vi "Sub_Online_FEA_Model.vi"(4 "Pin Location":i32, 11 "Modeling Parameters":T1) -> (2 "K Matrix":dbl[][](array[numeric]), 3 "M Matrix":dbl[][](array[numeric]))   [LabVIEW 2021]
panel:
  out "Element Length":dbl
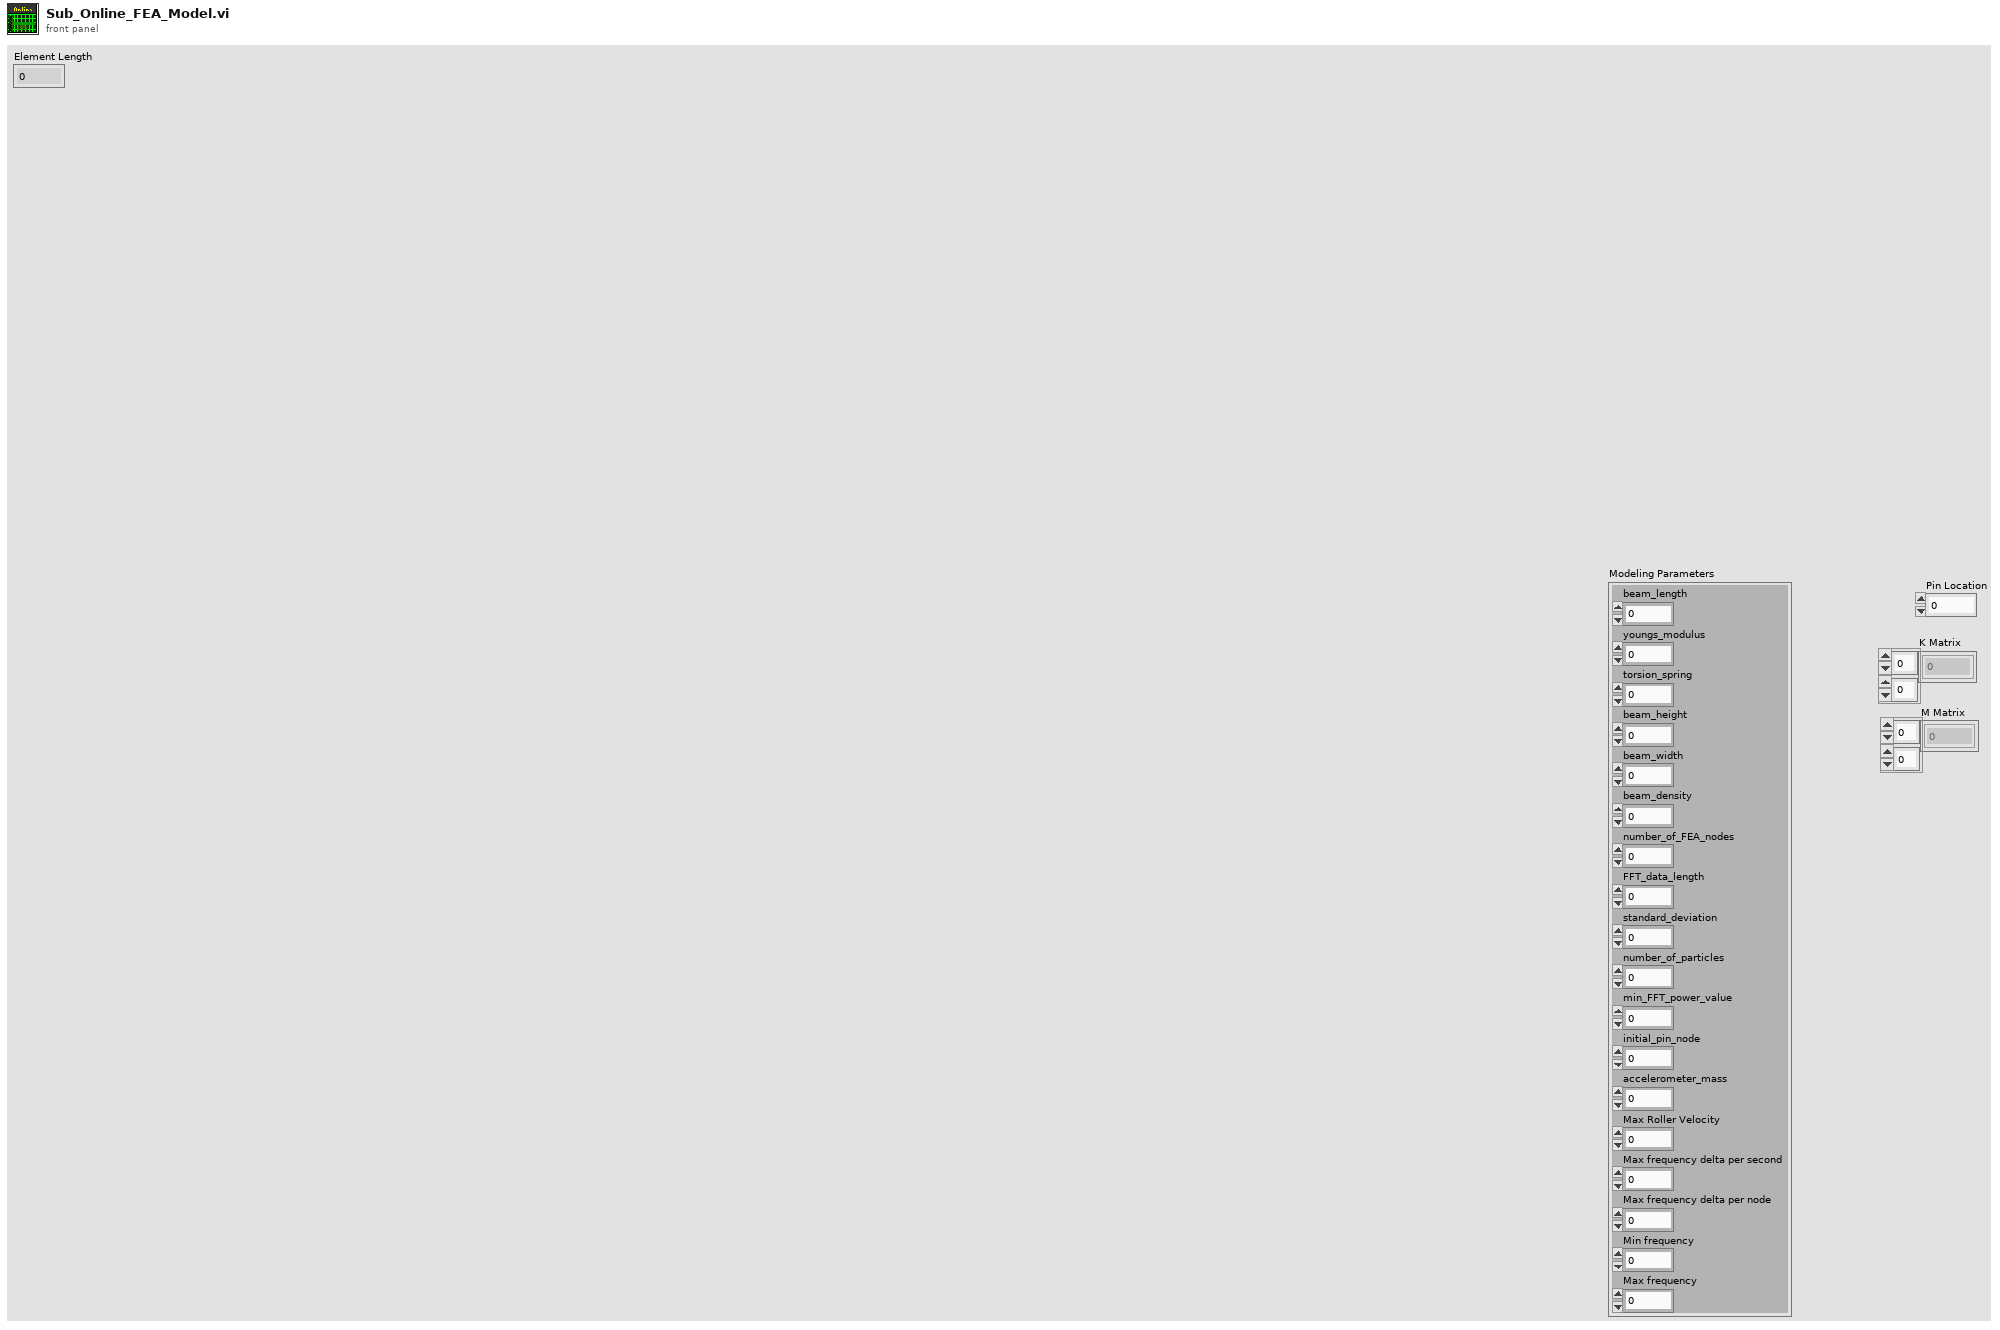
[diagram p1: front panel]
types:
  T1 = cluster{"beam_length":dbl, "youngs_modulus":dbl, "torsion_spring":dbl, "beam_height":dbl, "beam_width":dbl, "beam_density":dbl, "number_of_FEA_nodes":i32, "FFT_data_length":i32, "standard_deviation":dbl, "number_of_particles":i32, "min_FFT_power_value":dbl, "initial_pin_node":i32, "accelerometer_mass":dbl, "Max Roller Velocity":dbl, "Max frequency delta per second":dbl, "Max frequency delta per node":dbl, "Min frequency":dbl, "Max frequency":dbl}
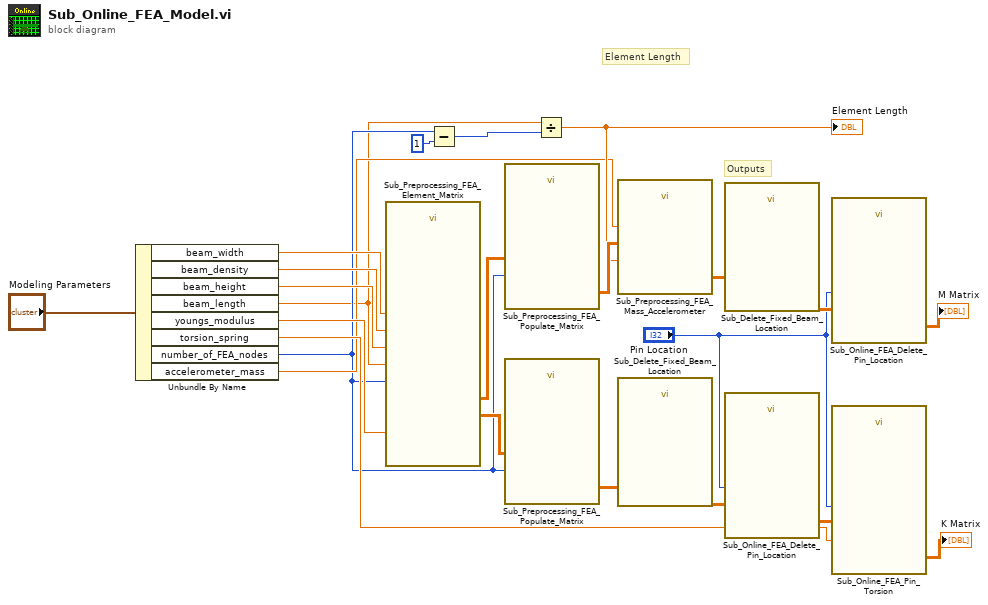
[diagram p0: block diagram]
diagram:
  # "Outputs"
  # "Element Length"
  n1 = Unbundle By Name("Modeling Parameters") -> ("beam_width"=w10:dbl, "beam_density"=w11:dbl, "beam_height"=w12:dbl, "beam_length"=w2:dbl, "youngs_modulus"=w13:dbl, "torsion_spring"=w14:dbl, "number_of_FEA_nodes"=w3:i32, "accelerometer_mass"=w4:dbl)
  n2 = call "Sub_Preprocessing_FEA_Element_Matrix.vi"("Length of Beam"=w2, "Young's Modulus"=w13, "No. of Nodes"=w3, "Height"=w12, "Width"=w10, "Density"=w11) -> ("M Element Matrix"=w16:dbl[][], "K Element Matrix"=w17:dbl[][])  [unwired: 11 in, 1 out]
  n3 = Subtract(x=w3, y=1) -> (x-y=w7:i32)
  n4 = call "Sub_Preprocessing_FEA_Populate_Matrix.vi"("No. of Nodes"=w3, "Element Matrix"=w16) -> ("Matrix w/o BC"=w8:dbl[][])  [unwired: 9 in]
  n5 = call "Sub_Preprocessing_FEA_Populate_Matrix.vi"("No. of Nodes"=w3, "Element Matrix"=w17) -> ("Matrix w/o BC"=w18:dbl[][])  [unwired: 9 in]
  n6 = Divide(x=w2, y=w7) -> (x/y=w5:dbl)
  "Element Length" <- w5
  n7 = call "Sub_Preprocessing_FEA_Mass_Accelerometer.vi"("Element Length"=w8, "accelerometer_mass"=w4, "Matrix w/o BC"=w5) -> ("Matrix W/ Accelerometer"=w9:dbl[][])  [unwired: 8 in]
  n8 = call "Sub_Delete_Fixed_Beam_Location.vi"("Pre-BC Matrix"=w18) -> ("Post-BC Matrix"=w20:dbl[][])  [unwired: 10 in]
  n9 = call "Sub_Delete_Fixed_Beam_Location.vi"("Pre-BC Matrix"=w9) -> ("Post-BC Matrix"=w19:dbl[][])  [unwired: 10 in]
  n10 = call "Sub_Online_FEA_Delete_Pin_Location.vi"("Pre-Pin Matrix"=w20, "Pin Location"="Pin Location") -> ("Post-Pin Matrix"=w21:dbl[][])  [unwired: 9 in]
  n11 = call "Sub_Online_FEA_Delete_Pin_Location.vi"("Pre-Pin Matrix"=w19, "Pin Location"="Pin Location") -> ("Post-Pin Matrix"=→"M Matrix":dbl[][])  [unwired: 9 in]
  n12 = call "Sub_Online_FEA_Pin_Torsion.vi"("Torsion"=w14, "Pin Location"="Pin Location", "K Matrix Input"=w21) -> ("K Matrix Output"=→"K Matrix":dbl[][])  [unwired: 8 in]
